vi "FE_PAB_OpenState.vi"(0 "FE":bool, 1 "XBPMX 2":dbl, 2 "XBPMY 2":dbl, 5 "Hutch":bool, 7 "PAB":bool, 9 "MGV":bool, 11 "FCV":bool) -> (4 "XBPMX 2":string, 6 "XBPMY 2":string)   [LabVIEW 2017]
panel:
  # "ORI num"
  # "SHOW state or value"
  # "um"
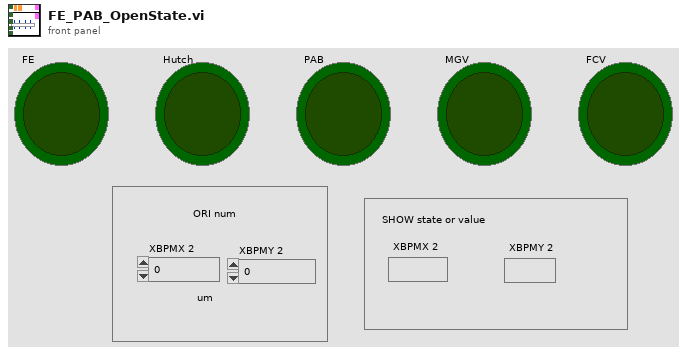
[diagram p1: front panel]
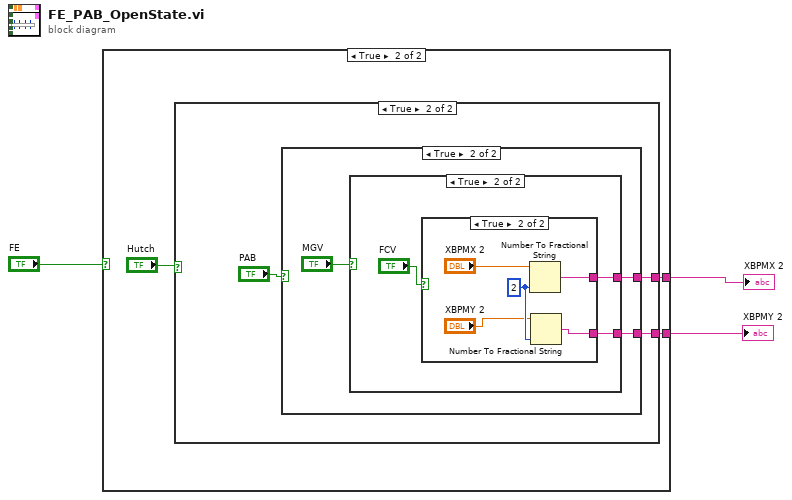
[diagram p0: block diagram]
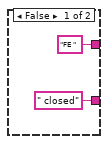
[diagram p2: hidden frame]
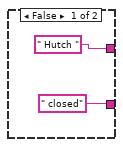
[diagram p3: hidden frame]
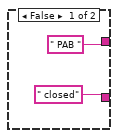
[diagram p4: hidden frame]
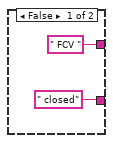
[diagram p5: hidden frame]
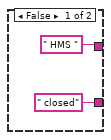
[diagram p6: hidden frame]
diagram:
  n1 = case shown="True" "FE" {
    tunnel: ["FE " w7] -> w2
    tunnel: [" closed" w6] -> w1
    frame False {
    }
    frame True {
      n2 = case shown="True" "Hutch" {
        tunnel: [" Hutch " w12] -> w7
        tunnel: [" closed" w11] -> w6
        frame False {
        }
        frame True {
          n3 = case shown="True" "PAB" {
            tunnel: [" PAB " w17] -> w12
            tunnel: [" closed" w16] -> w11
            frame False {
            }
            frame True {
              n4 = case shown="True" "MGV" {
                tunnel: [" FCV " w22] -> w17
                tunnel: [" closed" w21] -> w16
                frame False {
                }
                frame True {
                  n5 = case shown="True" "FCV" {
                    tunnel: [" HMS " w27] -> w22
                    tunnel: [" closed" w26] -> w21
                    frame False {
                    }
                    frame True {
                      w30 = i16 2 ("precision (6)")
                      n6 = Number To Fractional String(number="XBPMX 2", precision (6)=w30) -> (F-format string=w27:string)  [unwired: 2 in]
                      n7 = Number To Fractional String(number="XBPMY 2", precision (6)=w30) -> (F-format string=w26:string)  [unwired: 2 in]
                    }
                  }
                }
              }
            }
          }
        }
      }
    }
  }
  "XBPMX 2" <- w2
  "XBPMY 2" <- w1
